vi "Ch3_DoItYourself.vi"(9 "AM Wave Parameters":T2={"Signal Frequency"=500.0, "Modulation Frequency"=50.0, "Amplitude"=0.0}, 10 "Digitizing Parameters":T1={"Numbers of Samples"=100, "Sampling Frequency"=1000.0}) -> (2 "Waveform Output":cluster{"Displacement":dbl[], "Time":dbl[]})   [LabVIEW 2017]
uses:
  <vilib>/imath/engines/lvmath2/RunTimeEngine/Managers/WorkSpace/UID Generator.vi
  <vilib>/imath/engines/lvmath2/RunTimeEngine/RunTimeType/NIMS_RunTimeType_From StrictType (excl LVString).vi
  <instcachedir>/0/NIMS_RunTimeType_From StrictType (excl LVString)_1019F277F0A747EDBCA0F6C52CA54500.lvgen/NIMS_RunTimeType_From StrictType (excl LVString)_1019F277F0A747EDBCA0F6C52CA54500_000.vi
  <vilib>/imath/engines/lvmath2/RunTimeEngine/LocalVariableDefStatement/MC_LocalVariableDefStatement_Display.vi
  <vilib>/imath/engines/lvmath2/RunTimeEngine/RangeToken/NIMS_Range.vi
  <instcachedir>/0/NIMS_Range_69CB9AAD882742A19CF7E739BE79952C.lvgen/NIMS_Range_69CB9AAD882742A19CF7E739BE79952C_000.vi
  <vilib>/imathl/engines/lvmath/Functions/Error Handling/Create Error.vi
  <vilib>/imath/engines/lvmath2/RunTimeEngine/ArithmeticOperatorToken/NIMS_ArithmeticOperator_times.vi
  <instcachedir>/0/NIMS_ArithmeticOperator_times_9BECD6C28351466A83A029AF2762CD58.lvgen/NIMS_ArithmeticOperator_times_9BECD6C28351466A83A029AF2762CD58_000.vi
  <vilib>/imath/engines/lvmath2/RunTimeEngine/Managers/SymbolTable/Clear UID.vi
  <vilib>/imath/engines/lvmath2/RunTimeEngine/NodeEndStatement/NIMS_NodeEndStatement_Output.vi
  <instcachedir>/0/NIMS_NodeEndStatement_Output_53EC0D466D134D7ABD903AC30B43404B.lvgen/NIMS_NodeEndStatement_Output_53EC0D466D134D7ABD903AC30B43404B_005.vi
  <vilib>/imath/engines/lvmath2/RunTimeEngine/ErrorHandling/NIMS_Finalize Error.vi
  <vilib>/imath/engines/lvmath2/RunTimeEngine/Managers/SymbolTable/NIMS_WorkSpace.lvlib
panel:
  in  "Tab Control":enum32{"Page 1", "Page 2", "Page 3"}(tab)
  out "XY Graph":cluster{"t":dbl[], "x":dbl[]}(graph)
  in  "Initial Contraction Ratio":dbl=0.1
  in  "Max Contraction Ratio":dbl=0.3
  in  "One Cycle":dbl=10.0
  in  "BreakTime":dbl
  in  "Sampling Frequency2":dbl=1000.0
  out "XY Graph 2":cluster{"t1":dbl[], "lambda1":dbl[]}(graph)
  out "output array":dbl[](array[numeric])
  out "size(s)":i32
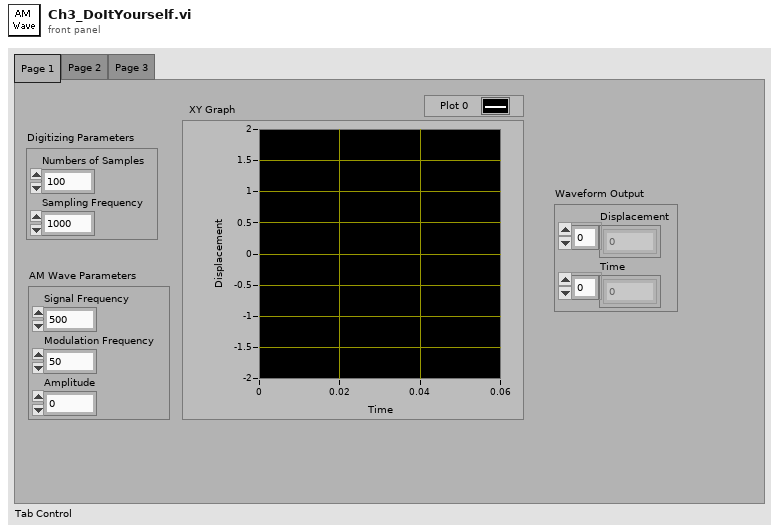
[diagram p1: front panel]
types:
  T1 = cluster{"Numbers of Samples":i32, "Sampling Frequency":dbl}
  T2 = cluster{"Signal Frequency":dbl, "Modulation Frequency":dbl, "Amplitude":dbl}
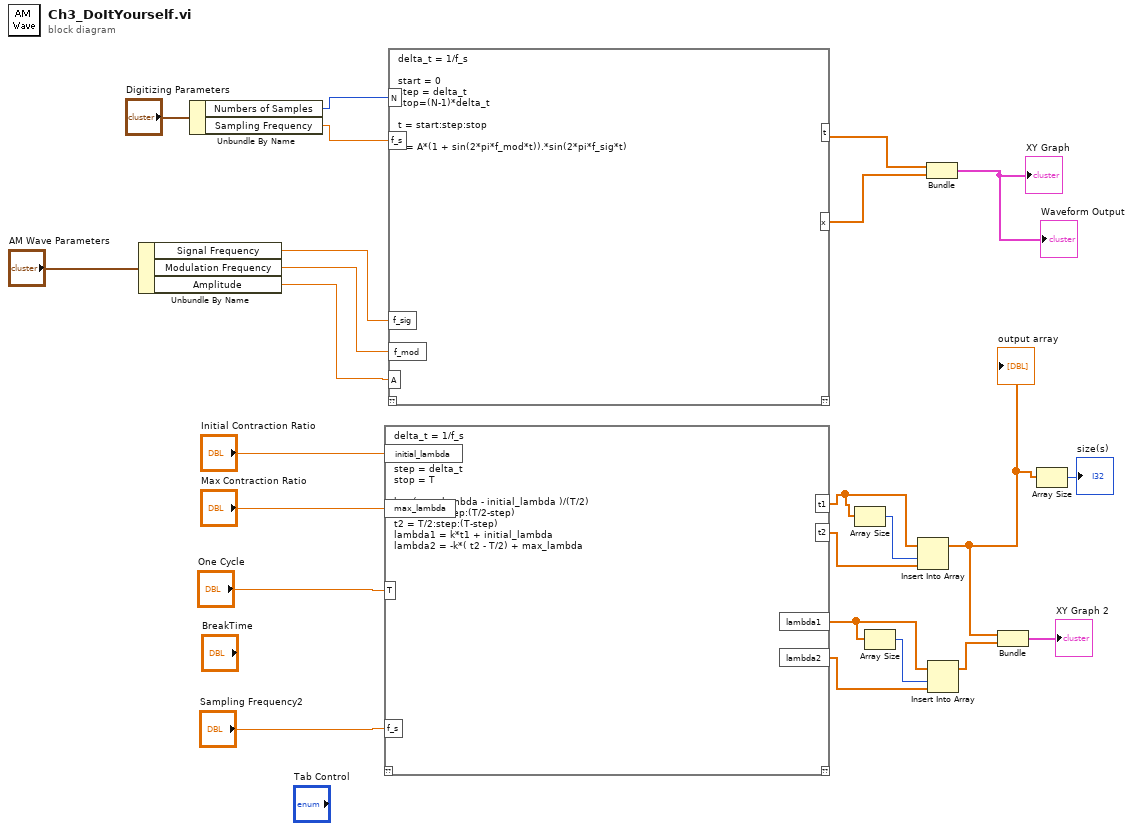
[diagram p0: block diagram]
diagram:
  n1 = Unbundle By Name("AM Wave Parameters") -> ("Signal Frequency"=w3:dbl, "Modulation Frequency"=w2:dbl, "Amplitude"=w1:dbl)
  n2 = Unbundle By Name("Digitizing Parameters") -> ("Numbers of Samples"=w7:i32, "Sampling Frequency"=w6:dbl)
  n3 = mathscript code="delta_t = 1/f_s\n\nstart = 0\nstep = delta_t\nstop = T\n\nk = (max_lambda - initial_lambda )/(T/2)\nt1 = start:step:(T/2-step)\nt2 = T/2:step:(T-step)\nlambda1 = k*t1 + initial_lambda\nlambda2 = -k*( t2 - T/2) + max_lambda"("initial_lambda"="Initial Contraction Ratio", "max_lambda"="Max Contraction Ratio", "T"="One Cycle", "f_s"="Sampling Frequency2") -> ("t1"=w18:dbl[], "t2"=w16:dbl[], "lambda1"=w13:dbl[], "lambda2"=w12:dbl[])  [unwired: 1 in, 1 out]
  n4 = mathscript code="delta_t = 1/f_s\n\nstart = 0\nstep = delta_t\nstop=(N-1)*delta_t\n\nt = start:step:stop\n\nx = A*(1 + sin(2*pi*f_mod*t)).*sin(2*pi*f_sig*t)"("N"=w7, "f_s"=w6, "A"=w1, "f_sig"=w3, "f_mod"=w2) -> ("t"=w24:dbl[], "x"=w23:dbl[])  [unwired: 1 in, 1 out]
  n5 = Array Size(array=w18) -> (size(s)=w17:i32)
  n6 = Array Size(array=w13) -> (size(s)=w14:i32)
  n7 = Insert Into Array(array=w18, index=w17, new element=w16) -> (w10:dbl[])
  "output array" <- w10
  n8 = Bundle("t"=w24, "x"=w23) -> (→"XY Graph" →"Waveform Output":cluster{"t":dbl[], "x":dbl[]})  [unwired: 1 in]
  n9 = Insert Into Array(array=w13, index=w14, new element=w12) -> (w11:dbl[])
  n10 = Bundle("t1"=w10, "lambda1"=w11) -> (→"XY Graph 2":cluster{"t1":dbl[], "lambda1":dbl[]})  [unwired: 1 in]
  n11 = Array Size(array=w10) -> (size(s)=→"size(s)":i32)
